vi "read metadata property.vi"(8 "error in":errorcluster, 10 "key":string, 11 "CEF_Configuration in":refnum<class "CEF_serializable configuration.lvclass">) -> (0 "error out":errorcluster, 1 "value":string, 2 "found":bool, 3 "CEF_Configuration out":refnum<class "CEF_serializable configuration.lvclass">)   [LabVIEW 2023, in "CEF.lvlib" / "CEF_serializable configuration.lvclass"]
doc: "Reads a single string property from the set of key/value pairs stored in the configuration class.Copyright 2017 National Instruments Corporation\n\nLicensed under the Apache License, Version 2.0 (the \"License\"); you may not use this file except in compliance with the License. You may obtain a copy of the License at http://www.apache.org/licenses/LICENSE-2.0\nUnless required by applicable law or agreed to in writing, software distributed under the License is distributed on an \"AS IS\" BASIS, WITHOUT WARRANTIES OR CONDITIONS OF ANY KIND, either express or implied. See the License for the specific language governing permissions and limitations under the License."
uses:
  CEF_serializable configuration.lvclass
  CEF_serializable configuration.lvclass/CEF_serializable configuration.ctl
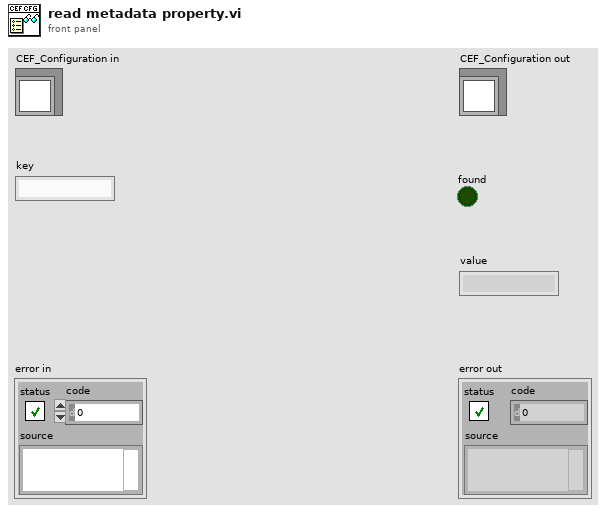
[diagram p1: front panel]
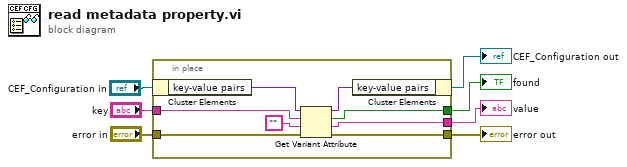
[diagram p0: block diagram]
diagram:
  n1 = in-place {
    in-place-border: "key" -> [w12]
    in-place-border: "error in" -> [w11]
    in-place-border: [w10] -> w3
    in-place-border: [w9] -> w2
    in-place-border: [w8] -> w1
    n2 = in-place-cluster #1("CEF_Configuration in") -> ("key-value pairs"=w15:variant)
    n3 = Get Variant Attribute(Variant=w15, name=w12, default value (empty Variant)="", error in=w11) -> (duplicate Variant=w14:variant, found=w8:bool, value=w9:string, error out=w10:errorcluster)
    n4 = in-place-cluster #1("key-value pairs"=w14) -> (→"CEF_Configuration out":refnum<class "CEF_serializable configuration.lvclass">)
  }
  "error out" <- w3
  "value" <- w2
  "found" <- w1
